vi "WPI_IMU_ADIS16448_WriteRegister.vi"(8 "error in (no error)":errorcluster, 9 "Data":u16=2049, 10 "ADIS16448 Register":T1=54 items=["SMPL_PRD"=54, "SENS_AVG"=56, "MSC_CTRL"=52, "ERROR_FLAGS"=60, "TEMP"=44, "BARO"=40, "Z_MAG"=36, "Y_MAG"=32, "X_MAG"=28, "Z_ACCEL"=24, "Y_ACCEL"=20, "X_ACCEL"=16, "Z_GYRO"=12, "Y_GYRO"=8, "X_GYRO"=4, "PID"=86], 11 "SPIDevRef in":T2) -> (0 "error out":errorcluster, 1 "Write OK?":bool, 2 "Register Value":u16, 3 "SPIDevRef out":T2)   [LabVIEW 2015, in "FRC ADI MXP IMU.lvlib"]
uses:
  FRC ADI MXP IMU.lvlib
  <vilib>/Rock Robotics/WPI/SPI/WPI_SPIDevRef.ctl
  <vilib>/Rock Robotics/SystemInterfaces/spilib/spi_bus.ctl
  WPI_IMU_ADIS16448_Registers.ctl
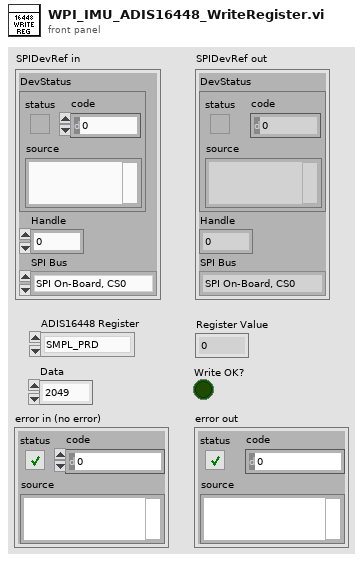
[diagram p1: front panel]
types:
  T1 = typedef "FRC ADI MXP IMU.lvlib/WPI_IMU_ADIS16448_Registers.ctl" = u8
  T2 = typedef "WPI_SPIDevRef.ctl" = cluster{"DevStatus":errorcluster, "Handle":i32, "SPI Bus":T3}
  T3 = typedef "spi_bus.ctl" = enum16{"SPI On-Board, CS0", "SPI On-Board, CS1", "SPI On-Board, CS2", "SPI On-Board, CS3", "SPI MXP", "Invalid"}
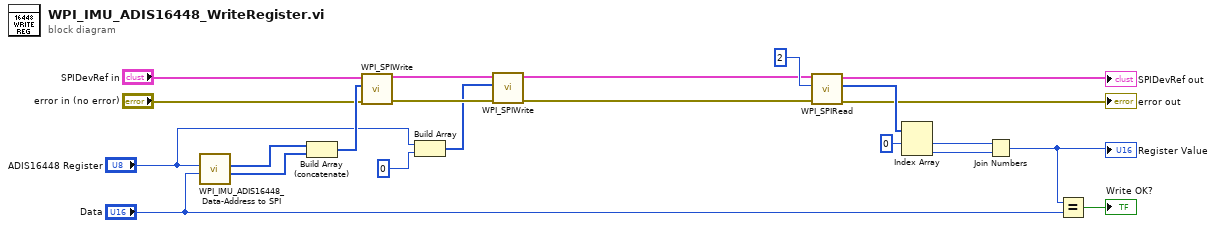
[diagram p0: block diagram]
diagram:
  n1 = call "WPI_IMU_ADIS16448_Data-Address to SPI.vi"("Data"="Data", "Address"="ADIS16448 Register") -> ("Low Word"=w15:u8[], "High Word"=w16:u8[])  [unwired: 8 in]
  n2 = Build Array (concatenate)(w16, w15) -> (w17:u8[])
  n3 = call <vilib>:"WPI_SPIWrite.vi"("error in (no error)"="error in (no error)", "Data To Send"=w17, "SPIDevRef"="SPIDevRef in") -> ("error out"=w13:errorcluster, "SPIDevRef"=w14:T2)  [unwired: 7 out]
  n4 = Build Array("ADIS16448 Register", 0) -> (w12:i32[])
  n5 = call <vilib>:"WPI_SPIWrite.vi"("error in (no error)"=w13, "Data To Send"=w12, "SPIDevRef"=w14) -> ("error out"=w1:errorcluster, "SPIDevRef"=w2:T2)  [unwired: 7 out]
  n6 = call <vilib>:"WPI_SPIRead.vi"("error in (no error)"=w1, "Num to Read"=2, "SPIDevRef"=w2) -> ("error out"=→"error out":errorcluster, "Received Data"=w20:u8[], "SPIDevRef"=→"SPIDevRef out":T2)  [unwired: 6 in]
  n7 = Index Array(array=w20, index #1=0 ("index")) -> (element #1=w9:u8, element #2=w8:u8)  [unwired: 1 in]
  n8 = Join Numbers(hi=w9, lo=w8) -> ((hi.lo)=w7:u16)
  "Register Value" <- w7
  n9 = Equal?(x=w7, y="Data") -> (x = y?=→"Write OK?":bool)
